vi "init-private-data.vi"(8 "error in (no error)":errorcluster, 11 "clone-id":i32) -> (0 "error out":errorcluster, 3 "module-data":T1)   [LabVIEW 2020, in "reporting-device.lvlib"]
uses:
  reporting-device.lvlib
  Module Data--cluster.ctl
  <userlib>/Zaphiro/GTools/Redis/Sources/Redis/Redis.lvclass
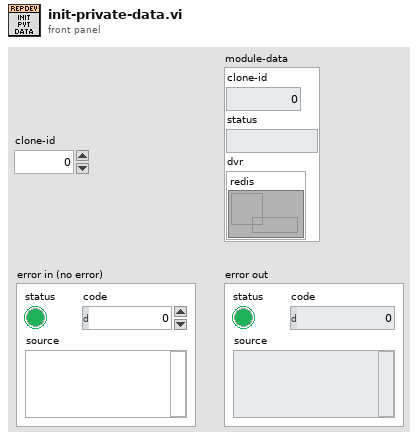
[diagram p1: front panel]
types:
  T1 = typedef "reporting-device.lvlib/Module Data--cluster.ctl" = cluster{"clone-id":i32, "status":string, "dvr":cluster{"redis":refnum<data-value>}}
  T2 = cluster{"output cluster":refnum<class "Redis.lvclass">}
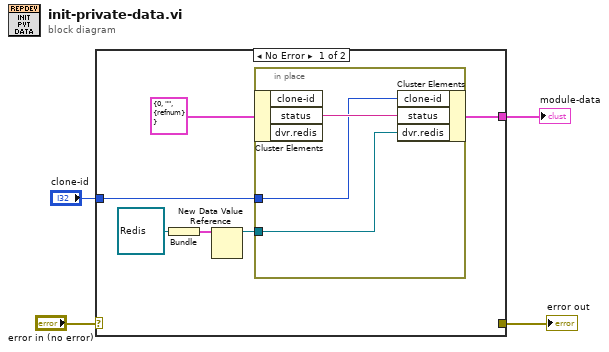
[diagram p0: block diagram]
diagram:
  n1 = case shown="No Error" "error in (no error)" {
    selector: "error in (no error)" -> [_ w14]
    tunnel: [w9 _] -> w2
    tunnel: [_ w14] -> w4
    tunnel: "clone-id" -> [w7 _]
    frame No Error {
      n2 = Bundle("output cluster"=refnum<class "Redis.lvclass"> refnum) -> (w6:T2)  [unwired: 1 in]
      n3 = New Data Value Reference(data value=w6) -> (data value reference=w8:refnum<data-value>)  [unwired: 1 in, 1 out]
      n4 = in-place {
        in-place-border: w8 -> [w12]
        in-place-border: w7 -> [w11]
        n5 = in-place-cluster #1(T1 {"clone-id"=0, "status"="", "dvr"={"redis"=refnum}} ("Data Cluster")) -> ("status"=w13:string)  [unwired: 2 out]
        n6 = in-place-cluster #1("clone-id"=w11, "status"=w13, "dvr.redis"=w12) -> (w9:T1)
      }
    }
    frame Error {
    }
  }
  "error out" <- w4
  "module-data" <- w2
